vi "Close Stream.vi"(8 "error in (no error)":errorcluster, 9 "Device Number":string, 10 "Stream Number (1)":u8=1, 11 "VISA resource name":refnum<visa-resource-name>) -> (0 "error out":errorcluster, 3 "VISA resource name out":refnum<visa-resource-name>)   [LabVIEW 2015, in "Zaber A Series.lvlib"]
doc: "Closes a stream, ending the ability to add new commands to it.\n\nUse the same stream number provided to the Open Stream VI - zero for the live stream, or a positive number for a saved stream buffer.\n\nLive streams are automatically erased when they are both closed and have finished executing. Buffered streams are saved in device memory and you must use the Erase Stream VI to remove them.\n\nThis VI does not check in advance for error conditions such as streams not being supported.\n\nThis VI requires that the Initialize VI has been called with the same serial port and that the specified stream is open."
uses:
  Zaber A Series.lvlib
  Private/All Commands.ctl
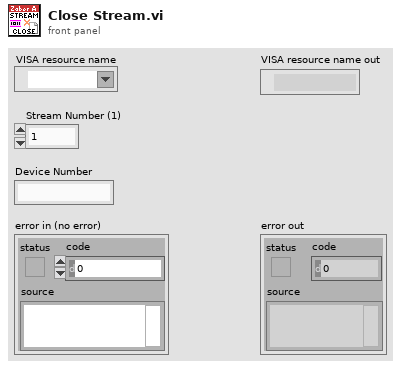
[diagram p1: front panel]
types:
  T1 = typedef "Zaber A Series.lvlib/All Commands.ctl" = string
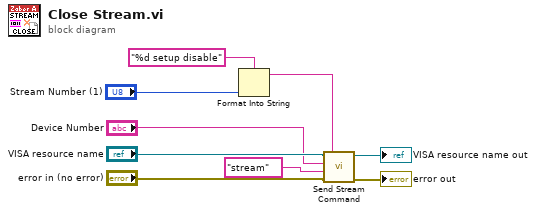
[diagram p0: block diagram]
diagram:
  n1 = Format Into String(format string="%d setup disable", "Stream Number (1)") -> (resulting string=w2:string)  [unwired: 2 in, 1 out]
  n2 = call "Send Stream Command.vi"("Data"=w2, "error in (no error)"="error in (no error)", "Command"=T1 "stream" ("Complete Command List"), "Device Number"="Device Number", "VISA resource name"="VISA resource name") -> ("error out"=→"error out":errorcluster, "VISA resource name out"=→"VISA resource name out":refnum<visa-resource-name>)  [unwired: 5 in]
